vi "Oriantation Problem Fix.vi"(1 "Oriantation Info Modified":T1, 2 "Oriantation Info Origianl":T1) -> (0 "Oriantation Info Fixed":T1)   [LabVIEW 2013]
panel:
  # "The Horizontal \nVector of the \nCamera Mounts\nDistance"
  # "The Horizontal \nVector of the \nCamera Mounts\nDistance"
  # "The Horizontal \nVector of the \nCamera Mounts\nDistance"
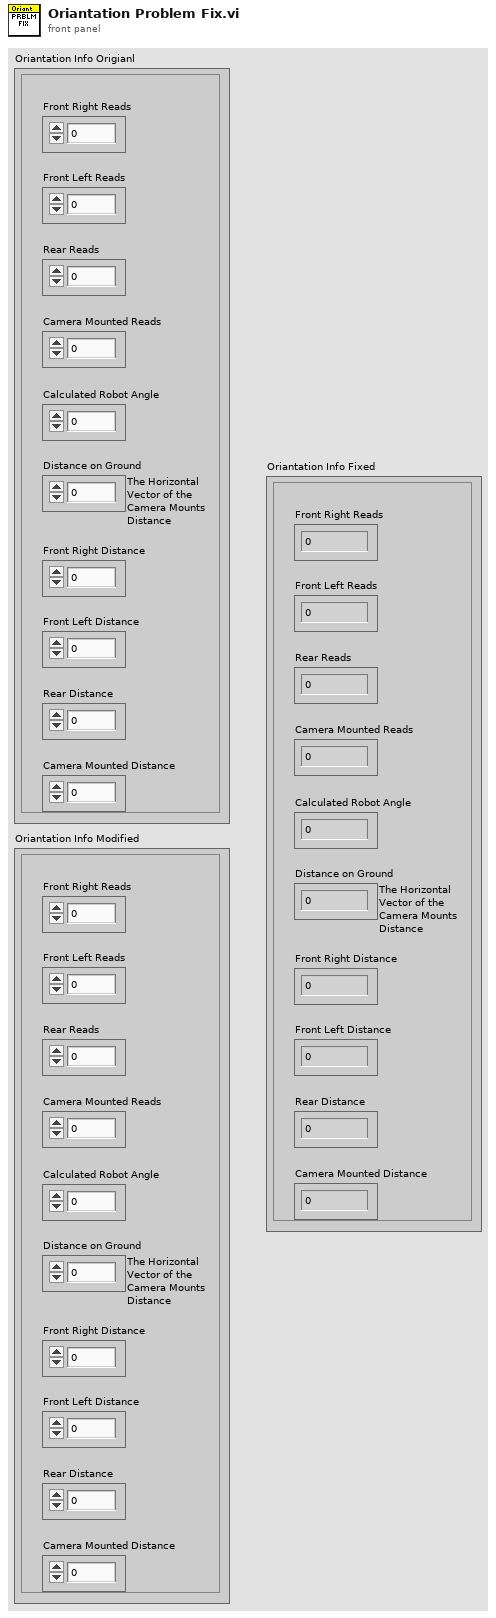
[diagram p1: front panel]
types:
  T1 = cluster{"Front Right Reads":dbl, "Front Left Reads ":dbl, "Rear Reads":dbl, "Camera Mounted Reads":dbl, "Calculated Robot Angle":dbl, "Distance on Ground":dbl, "Front Right Distance":dbl, "Front Left Distance":dbl, "Rear Distance":dbl, "Camera Mounted Distance":dbl}
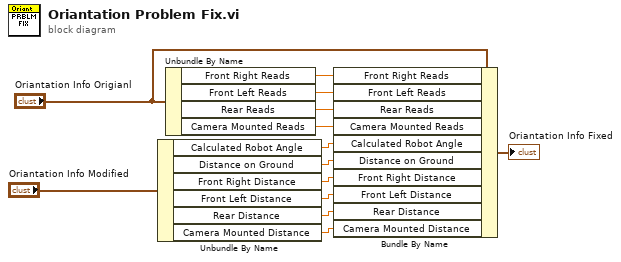
[diagram p0: block diagram]
diagram:
  n1 = Unbundle By Name("Oriantation Info Modified") -> ("Calculated Robot Angle"=w6:dbl, "Distance on Ground"=w5:dbl, "Front Right Distance"=w4:dbl, "Front Left Distance"=w3:dbl, "Rear Distance"=w2:dbl, "Camera Mounted Distance"=w1:dbl)
  n2 = Unbundle By Name("Oriantation Info Origianl") -> ("Front Right Reads"=w10:dbl, "Front Left Reads"=w9:dbl, "Rear Reads"=w8:dbl, "Camera Mounted Reads"=w7:dbl)
  n3 = Bundle By Name(cluster="Oriantation Info Origianl", "Front Right Reads"=w10, "Front Left Reads"=w9, "Rear Reads"=w8, "Camera Mounted Reads"=w7, "Calculated Robot Angle"=w6, "Distance on Ground"=w5, "Front Right Distance"=w4, "Front Left Distance"=w3, "Rear Distance"=w2, "Camera Mounted Distance"=w1) -> (→"Oriantation Info Fixed":T1)
